vi "CU_testClassifier.vi"(6 "DataTypes":T1=enum."Test Data", 8 "error in":errorcluster, 9 "Classifier Session Ref":T2, 10 "Indices":i8[](array[numeric]), 11 "ClassifierClass in":refnum<class "ClassifierClass.lvclass">) -> (0 "error out":errorcluster, 1 "Accuracy":dbl, 2 "Confusion Matrix":i32[][](array[numeric]), 3 "ClassifierClass out":refnum<class "ClassifierClass.lvclass">)   [LabVIEW 2016, in "Classifier.lvlib" / "ClassifierClass.lvclass"]
uses:
  ClassifierClass.lvclass
  <vilib>/vision/Classification.llb/IMAQ Classifier Session.ctl
  CU_DataTypes.ctl
  ClassifierClass.lvclass/ClassifierClass.ctl
  CU_CohenKappa.vi
  <vilib>/vision/NI_Vision_Development_Module.lvlib
  <vilib>/addons/Machine Learning/NILabs_MLT.lvlib
  Classifier.lvlib
panel:
  # "This VI is a part of BCI Design library, http://www.ru-bci.org \nCopyright © 2020, Sotnikov Peter, All rights reserved. License: CC BY-NC 4.0"
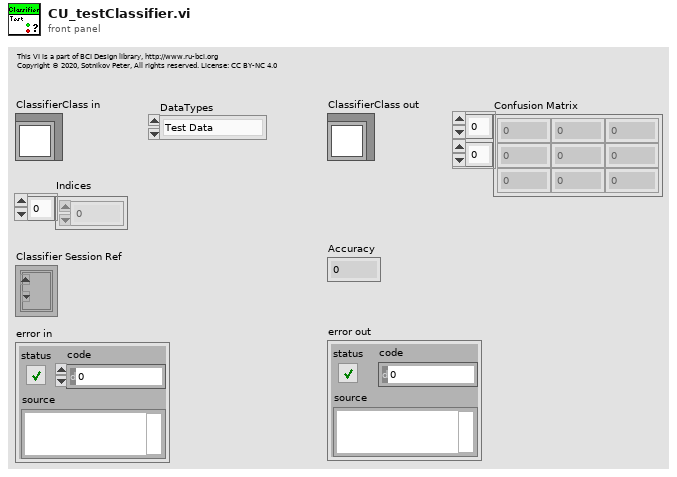
[diagram p1: front panel]
types:
  T1 = typedef "Classifier.lvlib/CU_DataTypes.ctl" = enum16{"Training Data", "Test Data", "Training Data (cross-check)", "Test Data (cross-check)"}
  T2 = typedef "IMAQ Classifier Session.ctl" = refnum<k1>
  T3 = typedef "XML_EEG_Features.lvlib/XML_FF_Trial.ctl" = cluster{"ClassLabel":string, "FeatureVector":dbl[]}
  T4 = typedef "Classifier.lvlib/CU_ClassifierQualityMeasure.ctl" = enum16{"Accuracy", "Cohen's kappa"}
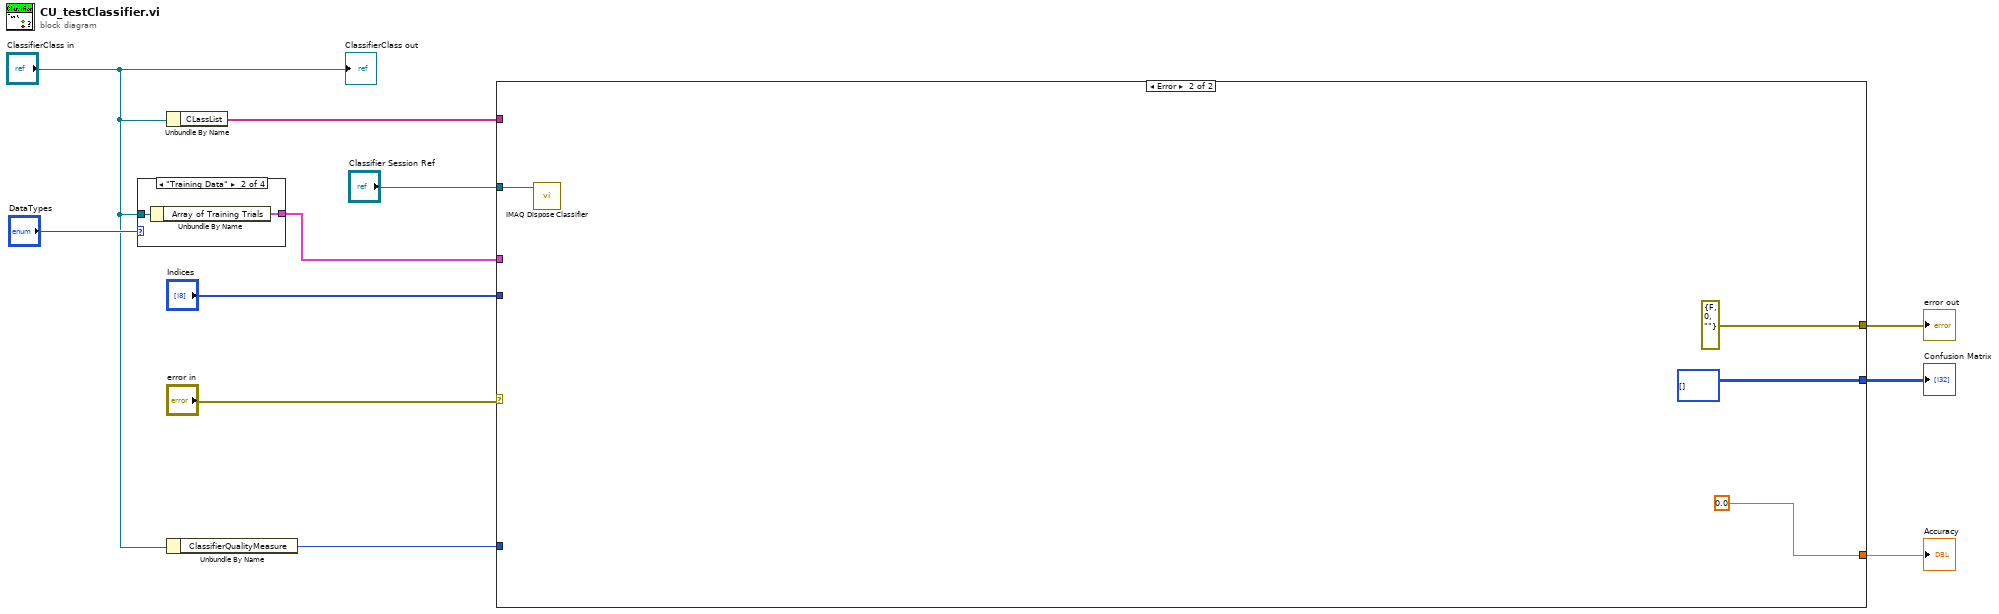
[diagram p0: block diagram]
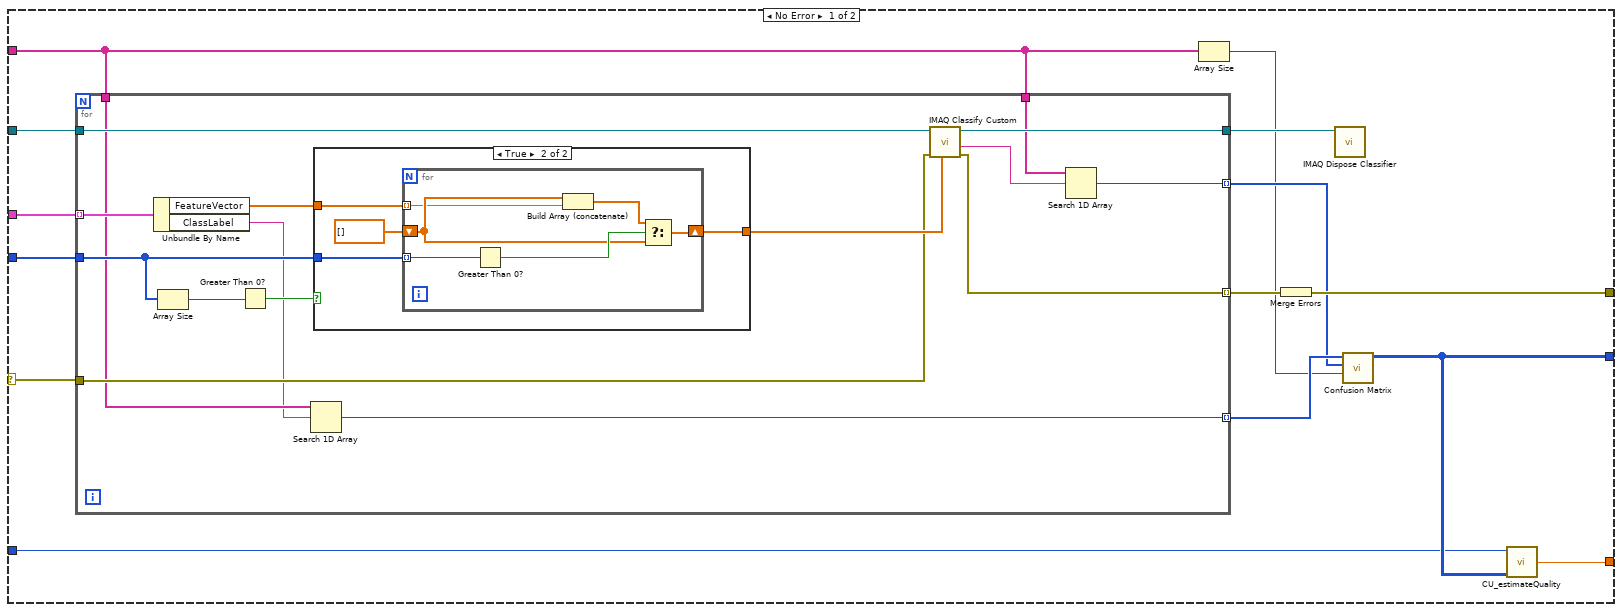
[diagram p2: hidden frame]
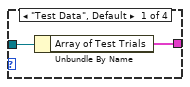
[diagram p4: hidden frame]
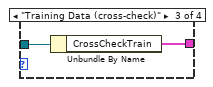
[diagram p5: hidden frame]
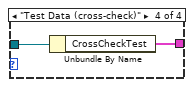
[diagram p6: hidden frame]
diagram:
  n1 = case shown="\"Training Data\"" "DataTypes" {
    tunnel: "ClassifierClass in" -> [w13 w15 w17 w19]
    tunnel: [w12 w14 w16 w18] -> w9
    frame "Test Data", Default {
      n2 = Unbundle By Name(w13) -> ("Array of Test Trials"=w12:T3[])
    }
    frame "Training Data" {
      n3 = Unbundle By Name(w15) -> ("Array of Training Trials"=w14:T3[])
    }
    frame "Training Data (cross-check)" {
      n4 = Unbundle By Name(w17) -> ("CrossCheckTrain"=w16:T3[])
    }
    frame "Test Data (cross-check)" {
      n5 = Unbundle By Name(w19) -> ("CrossCheckTest"=w18:T3[])
    }
  }
  n6 = Unbundle By Name("ClassifierClass in") -> ("CLassList"=w7:string[])
  n7 = Unbundle By Name("ClassifierClass in") -> ("ClassifierQualityMeasure"=w1:T4)
  n8 = case shown="Error" "error in" {
    selector: "error in" -> [w23 _]
    tunnel: [w33 errorcluster {"status"=FALSE, "code"=0, "source"=""} ("error IO")] -> w11
    tunnel: "Indices" -> [w32 _]
    tunnel: w9 -> [w29 _]
    tunnel: "Classifier Session Ref" -> [w28 w61]
    tunnel: w7 -> [w27 _]
    tunnel: [w22 0.0] -> w6
    tunnel: [w21 i32[][] [] ("Confusion Matrix")] -> w5
    tunnel: w1 -> [w20 _]
    frame No Error {
      n9 = for {
        tunnel: w28 -> [w44]
        tunnel: w29 -> [w47] mode=indexing
        tunnel: w32 -> [w45]
        tunnel: w23 -> [w42]
        tunnel: [w41] -> w31 mode=indexing
        tunnel: [w40] -> w30
        tunnel: w27 -> [w39]
        tunnel: w27 -> [w36]
        tunnel: [w37] -> w26 mode=indexing
        tunnel: [w34] -> w25 mode=indexing
        n10 = Unbundle By Name(w47) -> ("FeatureVector"=w46:dbl[], "ClassLabel"=w38:string)
        n11 = Array Size(array=w45) -> (size(s)=w49:i32)
        n12 = Greater Than 0?(x=w49) -> (x > 0?=w48:bool)
        n13 = Search 1D Array(1D array=w39, element=w38) -> (index of element=w37:i32)  [unwired: 1 in]
        n14 = case shown="True" w48 {
          tunnel: w46 -> [w50 w54]
          tunnel: w45 -> [_ w53]
          tunnel: [w50 w51] -> w43
          frame False {
          }
          frame True {
            n15 = for {
              tunnel: w54 -> [w56] mode=indexing
              tunnel: w53 -> [w60] mode=indexing
              shift-right: [w59] -> w51
              shift-left: dbl[] [] -> [w57]
              n16 = Greater Than 0?(x=w60) -> (x > 0?=w58:bool)
              n17 = Build Array (concatenate)(w57, w56) -> (w55:dbl[])
              n18 = Select(t=w55, s=w58, f=w57) -> (s? t:f=w59:dbl[])
            }
          }
        }
        n19 = call "IMAQ Classify Custom"("Feature Vector"=w43, "error in (no error)"=w42, "Classifier Session"=w44) -> ("error out"=w41:errorcluster, "Class"=w35:string, "Classifier Session (dup)"=w40:T2)  [unwired: 3 in, 3 out]
        n20 = Search 1D Array(1D array=w36, element=w35) -> (index of element=w34:i32)  [unwired: 1 in]
      }
      n21 = Array Size(array=w27) -> (size(s)=w24:i32)
      n22 = Merge Errors(w31) -> (w33:errorcluster)
      n23 = call "IMAQ Dispose Classifier"("Classifier Session"=w30) -> ()  [unwired: 10 in, 1 out]
      n24 = call <vilib>:"Confusion Matrix.vi"("# of classes"=w24, "Predicted class labels"=w25, "Actual class labels"=w26) -> ("Confusion Matrix"=w21:i32[][])  [unwired: 7 in, 1 out]
      n25 = call "CU_estimateQuality.vi"("Quality Measure in"=w20, "Confusion Matrix in"=w21) -> ("Classification Quality out"=w22:dbl)  [unwired: 6 in]
    }
    frame Error {
      n26 = call "IMAQ Dispose Classifier"("Classifier Session"=w61) -> ()  [unwired: 10 in, 1 out]
    }
  }
  "error out" <- w11
  "Accuracy" <- w6
  "Confusion Matrix" <- w5
  "ClassifierClass out" <- "ClassifierClass in"
